vi "SR2000从站数据和索引.vi"(9 "y":i32, 10 "x":i32, 11 "data out":string) -> (0 "颜色":u32, 1 "显示数据":string, 2 "索引列":i32, 3 "索引行":i32)   [LabVIEW 2011]
panel:
  out "数值":i32
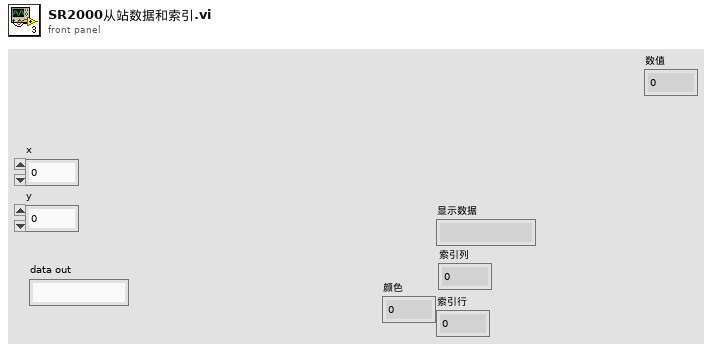
[diagram p1: front panel]
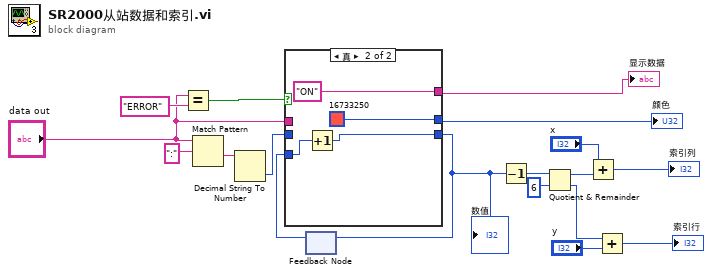
[diagram p0: block diagram]
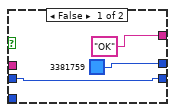
[diagram p2: hidden frame]
diagram:
  n1 = Equal?(x="data out", y="ERROR") -> (x = y?=w13:bool)
  n2 = Match Pattern(string="data out", regular expression=":" ("正则表达式")) -> (after substring=w18:string)  [unwired: 1 in, 3 out]
  n3 = Decimal String To Number(string=w18) -> (number=w15:i32)  [unwired: 2 in, 1 out]
  n4 = feedback #1() -> (w17:i32)  [unwired: 1 in]
  n5 = case shown="真" w13 {
    tunnel: ["OK" "ON"] -> w6
    tunnel: w15 -> [w19 _]
    tunnel: [w19 w23] -> w16
    tunnel: w17 -> [_ w24]
    tunnel: [u32 3381759 u32 16733250] -> w7
    tunnel: "data out" -> [_ _]
    frame False {
    }
    frame True {
      n6 = Increment(x=w24) -> (x+1=w23:i32)
    }
  }
  "显示数据" <- w6
  "颜色" <- w7
  "数值" <- w16
  n7 = feedback-in #1(w16) -> ()
  n8 = Decrement(x=w16) -> (x-1=w14:i32)
  n9 = Quotient & Remainder(x=w14, y=6) -> (x-y*floor(x/y)=w9:i32, floor(x/y)=w8:i32)
  n10 = Add(x="x", y=w9) -> (x+y=→"索引列":i32)
  n11 = Add(x=w8, y="y") -> (x+y=→"索引行":i32)
